vi "Fitter.vi"(8 "error in (no error)":errorcluster, 11 "CorrFactor in":refnum<class "CorrFactor.lvclass">) -> (0 "error out":errorcluster, 3 "CorrFactor out":refnum<class "CorrFactor.lvclass">)   [LabVIEW 2018, in "AnalysisPlugins.lvlib" / "CorrFactor.lvclass"]
uses:
  CorrFactor.lvclass
  C:/projects/ICDAS/NistPluggableModules/Analysis/AnalysisPlugins/AnalysisPluginBaseClass/AnalysisPluginsBase.lvclass
  AnalysisPluginBaseClass/AnalysisPluginsBase.lvclass/AnalysisPluginsBase.ctl
  FitterBaseClass/Typedefs/clAnalysisConfig.ctl
  Typedefs/FitterResult.ctl
  CorrFactor.lvclass/CorrFactor.ctl
  AnalysisPluginBaseClass/Accessors/Read DelayCorr.vi
  AnalysisPluginBaseClass/Accessors/Read MagCorr.vi
  AnalysisPluginBaseClass/Accessors/Read AnalysisConfig.vi
  Accessors/Read Function.vi
  AnalysisPluginBaseClass/Accessors/Write Result.vi
  AnalysisPluginBaseClass/Accessors/Read Window.vi
  FGen/MemberClasses/FunctionBaseClass/FunctionBase.lvclass
  FitterBaseClass/FitterBase.lvclass
panel:
  out "Phase (rad)":dbl[](array[numeric])
  out "Magnitude":dbl[](array[numeric])
  out "Waveform Graph":dbl[][](graph)
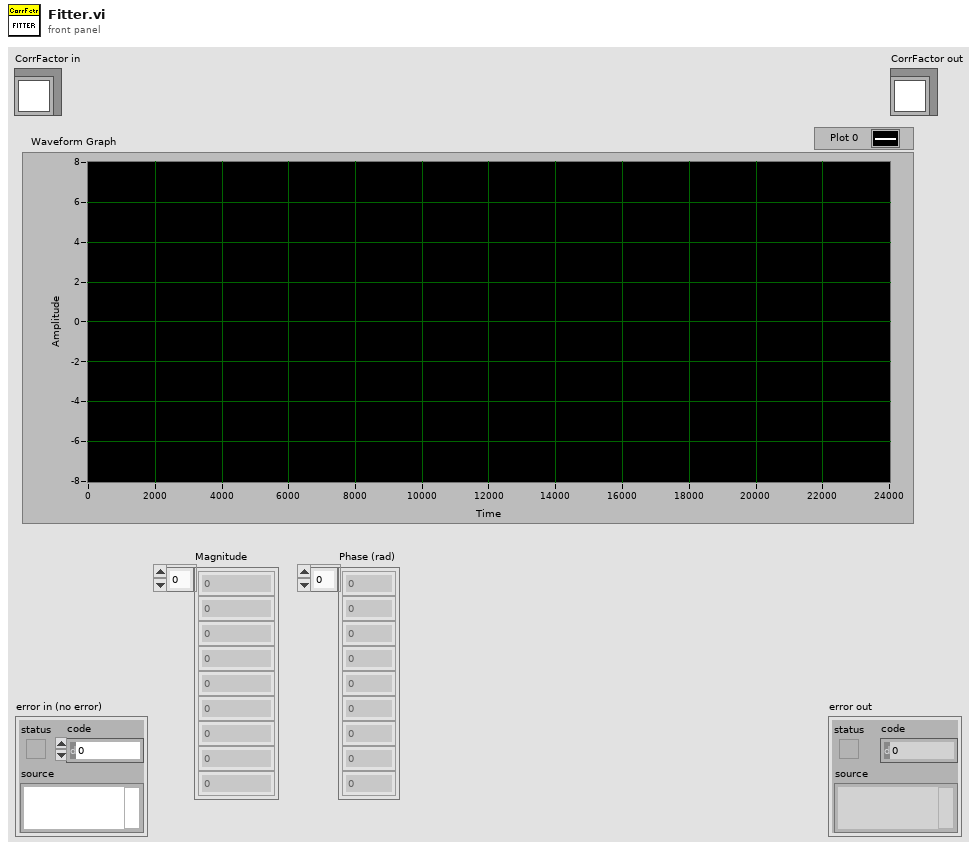
[diagram p1: front panel]
types:
  T1 = typedef "AnalysisPlugins.lvlib/CorrFactor.lvclass/FitterResult.ctl" = cluster{"Synx":cdb[], "Freq":dbl, "ROCOF":dbl}
  T2 = typedef "AnalysisPlugins.lvlib/FitterBase.lvclass/clAnalysisConfig.ctl" = cluster{"F0":u32, "SettlingTime":dbl, "AnalysisCycles":dbl, "SampleRate":dbl, "NumChannels":u32, "TsOffset":enum16{"start", "middle", "end"}}
  T3 = typedef "AnalysisPlugins.lvlib/AnalysisPluginsBase.lvclass/clWindowData.ctl" = cluster{"Timestamp":ext, "Samples":dbl[][], "Window Valid":bool, "T0":ext}
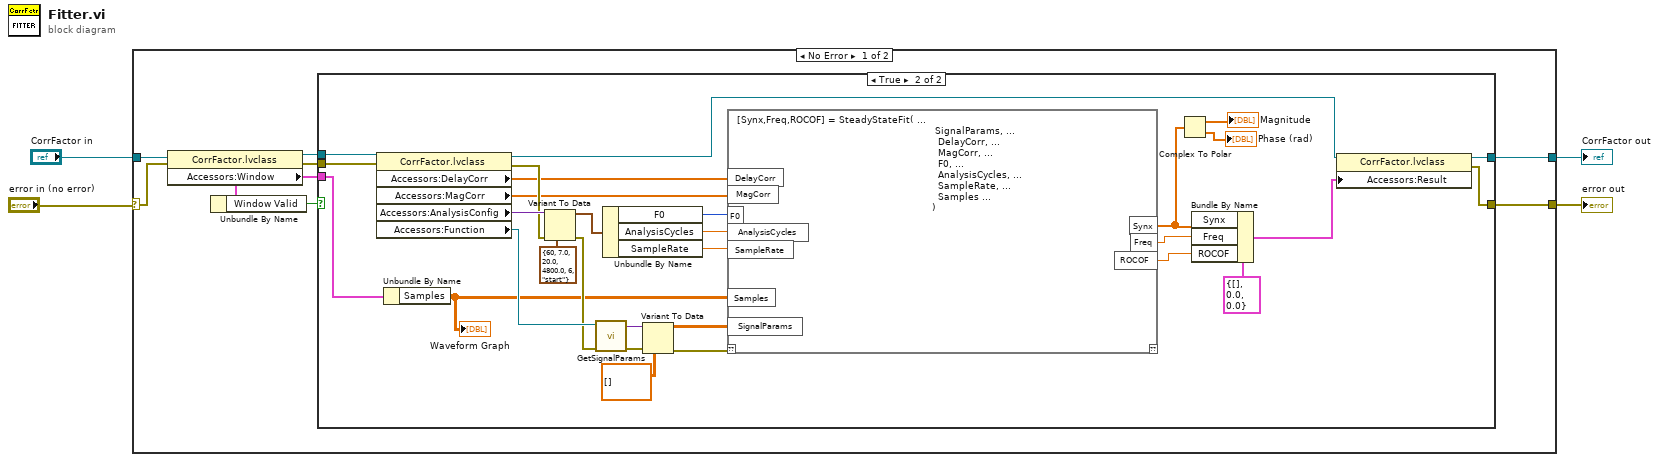
[diagram p0: block diagram]
diagram:
  n1 = case shown="No Error" "error in (no error)" {
    selector: "error in (no error)" -> [w11 w45]
    tunnel: "CorrFactor in" -> [w12 w46]
    tunnel: [w6 w46] -> w2
    tunnel: [w5 w45] -> w1
    frame No Error {
      n2 = property class="CorrFactor.lvclass"(reference=w12, error in=w11) -> (reference out=w8:refnum<class "CorrFactor.lvclass">, error out=w7:errorcluster, "Accessors:Window"=w9:T3)
      n3 = Unbundle By Name(w9) -> ("Window Valid"=w10:bool)
      n4 = case shown="True" w10 {
        tunnel: w9 -> [_ w42]
        tunnel: w8 -> [w14 w44]
        tunnel: w7 -> [w13 w43]
        tunnel: [w14 w17] -> w6
        tunnel: [w13 w16] -> w5
        frame False {
        }
        frame True {
          n5 = property class="CorrFactor.lvclass"(reference=w44, error in=w43) -> (reference out=w24:refnum<class "CorrFactor.lvclass">, error out=w35:errorcluster, "Accessors:DelayCorr"=w32:dbl[], "Accessors:MagCorr"=w31:dbl[], "Accessors:AnalysisConfig"=w36:variant, "Accessors:Function"=w38:refnum<class "FunctionBase.lvclass">)
          n6 = Unbundle By Name(w42) -> ("Samples"=w26:dbl[][])
          "Waveform Graph" <- w26
          n7 = Variant To Data(error in=w35, type=T2 {"F0"=60, "SettlingTime"=7.0, "AnalysisCycles"=20.0, "SampleRate"=4800.0, "NumChannels"=6, "TsOffset"=enum."start"} ("clAnalysisConfig"), Variant=w36) -> (data=w33:T2, error out=w34:errorcluster)
          n8 = call-dynamic "GetSignalParams.vi"("error in (no error)"=w34, "FunctionBase in"=w38) -> ("error out"=w41:errorcluster, "Params"=w40:variant)  [unwired: 7 in, 1 out]
          n9 = Unbundle By Name(w33) -> ("F0"=w30:u32, "AnalysisCycles"=w29:dbl, "SampleRate"=w28:dbl)
          n10 = Variant To Data(error in=w41, type=dbl[][] [], Variant=w40) -> (data=w27:dbl[][], error out=w25:errorcluster)
          n11 = script code="[Synx,Freq,ROCOF] = SteadyStateFit( ...\n                                                                  SignalParams, ...\n                                                                   DelayCorr, ...\n                                                                   MagCorr, ...\n                                                                   F0, ...\n                                                                   AnalysisCycles, ...\n                                                                   SampleRate, ...\n                                                                   Samples ...\n                                                                 )"("??"=w25, "SignalParams"=w27, "DelayCorr"=w32, "MagCorr"=w31, "F0"=w30, "AnalysisCycles"=w29, "SampleRate"=w28, "Samples"=w26) -> ("Synx"=w20:cdb[], "Freq"=w23:dbl, "ROCOF"=w22:dbl)  [unwired: 1 out]
          n12 = Complex To Polar(r * e^(i*theta)=w20) -> (r=→"Magnitude":dbl[], theta=→"Phase (rad)":dbl[])
          n13 = Bundle By Name(cluster=T1 {"Synx"=[], "Freq"=0.0, "ROCOF"=0.0} ("Fitter_Result"), "Synx"=w20, "Freq"=w23, "ROCOF"=w22) -> (w21:T1)
          n14 = property class="CorrFactor.lvclass"(reference=w24, "Accessors:Result"=w21) -> (reference out=w17:refnum<class "CorrFactor.lvclass">, error out=w16:errorcluster)  [unwired: 1 in]
        }
      }
    }
    frame Error {
    }
  }
  "error out" <- w1
  "CorrFactor out" <- w2
